vi "cm-pixel(SubVI).vi"(11 "NavData Out in":T1) -> (3 "cm per pixel":sgl format="%.2f")   [LabVIEW 2014]
uses:
  <vilib>/LVH/AR Drone Toolkit/Decode NavData/Typedefs/NavData Demo.ctl
  <vilib>/LVH/AR Drone Toolkit/AR Drone.lvlib
panel:
  in  "y":sgl=10.0
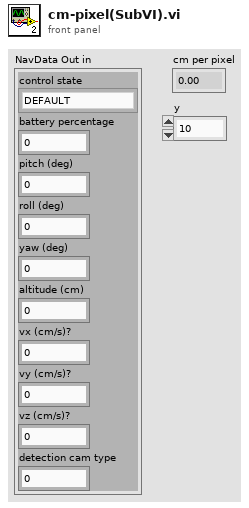
[diagram p1: front panel]
types:
  T1 = typedef "AR Drone.lvlib/NavData Demo.ctl" = cluster{"control state":enum32{"DEFAULT", "INIT", "LANDING", "FLYING", "HOVERING", "TEST", "TRANS_TAKEOFF", "TRANS_GOTOFIX", "TRANS_LANDING"}, "battery percentage":u32, "pitch (deg)":sgl, "roll (deg)":sgl, "yaw (deg)":sgl, "altitude (cm)":u32, "vx (cm/s)?":sgl, "vy (cm/s)?":sgl, "vz (cm/s)?":sgl, "detection cam type":u32}
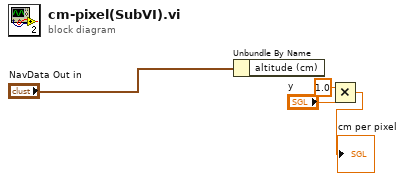
[diagram p0: block diagram]
diagram:
  n1 = Unbundle By Name("NavData Out in") -> ()  [unwired: 1 out]
  n2 = Multiply(x=sgl 1.0, y="y") -> (x*y=→"cm per pixel":sgl)
